vi "qKLC.vi"(0 "System no.":i32=1 min=1 max=4 step=1, 2 "Name":string, 3 "Name 2":string, 5 "error in":errorcluster, 6 "Item":string, 7 "Item 2":string) -> (14 "Response":string, 19 "error out":errorcluster)   [LabVIEW 2026]
doc: "Returns parameters of available Work/Tool combinations. The returned information depends on the used arguments. Applicable parameters are: name of Work coordinate system, name of Tool coordinate system, NLM, PLM, SSL, and SST. Name 2 is only valid in combination with Name; Item is only valid in combination with Name and Name 2; Item 2 is only valid in combination with Name, Name 2 and Item.\n\nC-887, F-206, M-8X0: Only for GCS syntax version = GCS 2.0 or higher (Check with CSV?.vi. If CSV?.vi is not supported, syntax version is GCS 1.0)."
panel:
  # "Returns parameters of available Work/Tool combinations. \nThe returned information depends on the used arguments."
  # "Only valid in combination\nwith Name:"
  # "Only valid in combination\nwith Name + Name 2:"
  # "Only valid in combination\nwith Name + Name 2 + Item:"
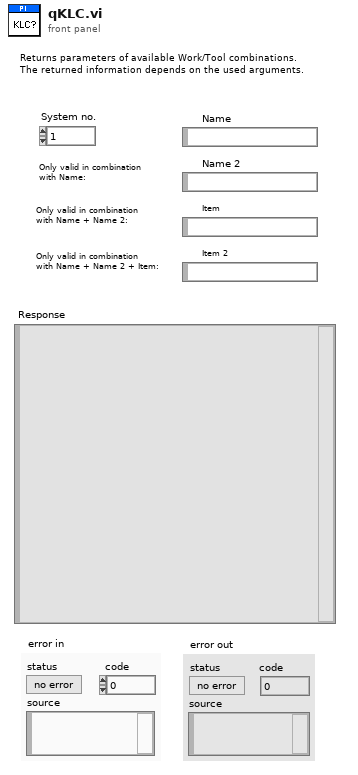
[diagram p1: front panel]
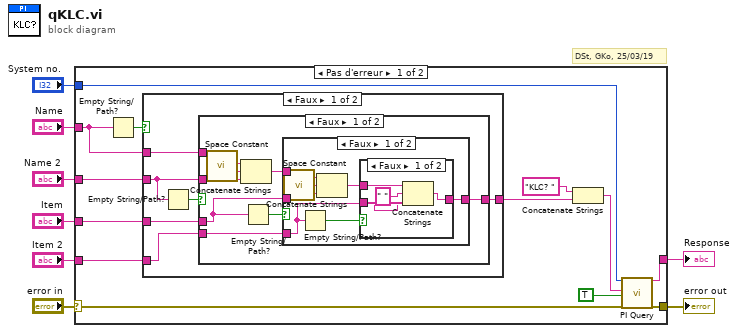
[diagram p0: block diagram]
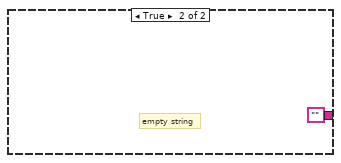
[diagram p5: hidden frame]
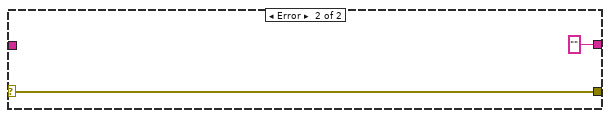
[diagram p6: hidden frame]
diagram:
  # "DSt, GKo, 25/03/19"
  n1 = case shown="Pas d'erreur" "error in" {
    selector: "error in" -> [w13 w51]
    tunnel: [w12 "" ("String read")] -> w8
    tunnel: [w11 w51] -> w7
    tunnel: "System no." -> [w21 _]
    tunnel: "Name" -> [w10 _]
    tunnel: "Name 2" -> [w18 _]
    tunnel: "Item" -> [w17 _]
    tunnel: "Item 2" -> [w16 _]
    frame No Error {
      n2 = Empty String/Path?(string/path=w10) -> (empty?=w9:bool)
      n3 = case shown="Faux" w9 {
        tunnel: w18 -> [w23 _]
        tunnel: w17 -> [w27 _]
        tunnel: w16 -> [w26 _]
        tunnel: [w25 ""] -> w15
        tunnel: w10 -> [w24 _]
        frame False {
          n4 = Empty String/Path?(string/path=w23) -> (empty?=w22:bool)
          n5 = case shown="Faux" w22 {
            tunnel: w27 -> [w29 _]
            tunnel: w26 -> [w35 _]
            tunnel: [w34 w49] -> w25
            tunnel: w24 -> [w33 w49]
            tunnel: w23 -> [w30 _]
            frame False {
              n6 = call <vilib>:"Space Constant.vi"() -> ("String"=w31:string)
              n7 = Concatenate Strings(w33, w31, w30) -> (w32:string)
              n8 = Empty String/Path?(string/path=w29) -> (empty?=w28:bool)
              n9 = case shown="Faux" w28 {
                tunnel: [w42 w48] -> w34
                tunnel: w35 -> [w37 _]
                tunnel: w32 -> [w41 w48]
                tunnel: w29 -> [w39 _]
                frame False {
                  n10 = call <vilib>:"Space Constant.vi"() -> ("String"=w40:string)
                  n11 = Empty String/Path?(string/path=w37) -> (empty?=w36:bool)
                  n12 = Concatenate Strings(w41, w40, w39) -> (w38:string)
                  n13 = case shown="Faux" w36 {
                    tunnel: [w46 w47] -> w42
                    tunnel: w38 -> [w45 w47]
                    tunnel: w37 -> [w43 _]
                    frame False {
                      n14 = Concatenate Strings(w45, " " ("string"), w43) -> (w46:string)
                    }
                    frame True {
                      # "empty string"
                    }
                  }
                }
                frame True {
                  # "empty string"
                }
              }
            }
            frame True {
              # "empty string"
            }
          }
        }
        frame True {
          # "empty string"
        }
      }
      n15 = Concatenate Strings("KLC? " ("string"), w15) -> (w19:string)
      n16 = call "PI Query.vi"("System no."=w21, "String to send"=w19, "Attach termination char.?"=TRUE ("Attach Linefeed?"), "error in"=w13) -> ("String read"=w12:string, "error out"=w11:errorcluster)  [unwired: 3 in, 11 out]
    }
    frame Error {
    }
  }
  "Response" <- w8
  "error out" <- w7
